vi "RPL_Top_Level_GUI.vi"() -> ()   [LabVIEW 2021]
uses:
  <vilib>/Utility/file.llb/Read Delimited Spreadsheet (string).vi
panel:
  out "Array":string[][](array[string])
  out "subarray":string[](array[string])
  in  "?":bool
  in  "Absolute Change":dbl
  out "ABORT\nACTIVATED":bool
  out "% Change":dbl[](array[numeric])
  in  "% Change":dbl
  out "all rows 2":string[][](array[string])
  in  "Fire Button":bool
  out "IGNITION":bool
  out "DEADMAN\nSWITCH":bool
  in  "Arm Button":bool
  out "POWER DISCONNECTED":bool
  in  "?":bool
  in  "SV6":bool
  in  "SV5":bool
  in  "SV4":bool
  in  "?":bool
  in  "SV3":bool
  in  "SV2":bool
  in  "SV1":bool
  in  "SV0":bool
  in  "GUITabs":T1(tab) caption="Tab Control"
  in  "Deadman Switch Pin":u16(ring) items=["FIO0", "FIO1", "FIO2", "FIO3", "FIO4", "FIO5", "FIO6", "FIO7", "EIO0", "EIO1", "EIO2", "EIO3", "EIO4", "EIO5", "EIO6", "EIO7", "CIO0", "CIO1", "CIO2", "CIO3", "MIO0", "MIO1", "MIO2"]
  in  "Solenoid Supply Pin":u16=5
  in  "LabJack Supply Pin":u16=7
  in  "Relay Supply Pin":u16=9
  in  "Igniter Pin":u16(ring)=7 items=["FIO0", "FIO1", "FIO2", "FIO3", "FIO4", "FIO5", "FIO6", "FIO7", "EIO0", "EIO1", "EIO2", "EIO3", "EIO4", "EIO5", "EIO6", "EIO7", "CIO0", "CIO1", "CIO2", "CIO3", "MIO0", "MIO1", "MIO2"]
  in  "LabJack IP Address":string="192.168.1.199"
  in  "LabJack Connection Type":u16(ring) items=["USB", "Ethernet"]
  in  "S: NO/NC":bool=TRUE
  in  "SV0 Pin":u16(ring)=8 items=["FIO0", "FIO1", "FIO2", "FIO3", "FIO4", "FIO5", "FIO6", "FIO7", "EIO0", "EIO1", "EIO2", "EIO3", "EIO4", "EIO5", "EIO6", "EIO7", "CIO0", "CIO1", "CIO2", "CIO3", "MIO0", "MIO1", "MIO2"]
  in  "SV1 Pin":u16(ring)=9 items=["FIO0", "FIO1", "FIO2", "FIO3", "FIO4", "FIO5", "FIO6", "FIO7", "EIO0", "EIO1", "EIO2", "EIO3", "EIO4", "EIO5", "EIO6", "EIO7", "CIO0", "CIO1", "CIO2", "CIO3", "MIO0", "MIO1", "MIO2"]
  in  "SV3 Pin":u16(ring)=11 items=["FIO0", "FIO1", "FIO2", "FIO3", "FIO4", "FIO5", "FIO6", "FIO7", "EIO0", "EIO1", "EIO2", "EIO3", "EIO4", "EIO5", "EIO6", "EIO7", "CIO0", "CIO1", "CIO2", "CIO3", "MIO0", "MIO1", "MIO2"]
  in  "SV2 Pin":u16(ring)=10 items=["FIO0", "FIO1", "FIO2", "FIO3", "FIO4", "FIO5", "FIO6", "FIO7", "EIO0", "EIO1", "EIO2", "EIO3", "EIO4", "EIO5", "EIO6", "EIO7", "CIO0", "CIO1", "CIO2", "CIO3", "MIO0", "MIO1", "MIO2"]
  in  "SV6 Pin":u16(ring)=14 items=["FIO0", "FIO1", "FIO2", "FIO3", "FIO4", "FIO5", "FIO6", "FIO7", "EIO0", "EIO1", "EIO2", "EIO3", "EIO4", "EIO5", "EIO6", "EIO7", "CIO0", "CIO1", "CIO2", "CIO3", "MIO0", "MIO1", "MIO2"]
  in  "SV5 Pin":u16(ring)=13 items=["FIO0", "FIO1", "FIO2", "FIO3", "FIO4", "FIO5", "FIO6", "FIO7", "EIO0", "EIO1", "EIO2", "EIO3", "EIO4", "EIO5", "EIO6", "EIO7", "CIO0", "CIO1", "CIO2", "CIO3", "MIO0", "MIO1", "MIO2"]
  in  "SV4 Pin":u16(ring)=12 items=["FIO0", "FIO1", "FIO2", "FIO3", "FIO4", "FIO5", "FIO6", "FIO7", "EIO0", "EIO1", "EIO2", "EIO3", "EIO4", "EIO5", "EIO6", "EIO7", "CIO0", "CIO1", "CIO2", "CIO3", "MIO0", "MIO1", "MIO2"]
  in  "S: NO/NC":bool=TRUE
  in  "S: NO/NC":bool=TRUE
  in  "S: NO/NC":bool=TRUE
  in  "S: NO/NC":bool=TRUE
  in  "S: NO/NC":bool=TRUE
  in  "S: NO/NC":bool=TRUE
  in  "R: NC/NO":bool=TRUE
  in  "R: NC/NO":bool=TRUE
  in  "R: NC/NO":bool=TRUE
  in  "R: NC/NO":bool=TRUE
  in  "R: NC/NO":bool=TRUE
  in  "R: NC/NO":bool=TRUE
  in  "R: NC/NO":bool=TRUE
  in  "TC1 Type":u16(ring)=7 items=["B", "E", "J", "K", "N", "R", "S", "T"]
  in  "TC2 Type":u16(ring)=3 items=["B", "E", "J", "K", "N", "R", "S", "T"]
  in  "TC1 +Channel":u16
  in  "TC2 -Channel":u16=3
  in  "TC2 +Channel":u16=2
  in  "TC1 -Channel":u16=1
  in  "PT2 Pin":u16=6
  in  "PT1 Pin":u16=8
  in  "PT3 Pin":u16=4
  in  "LP1 Pin":u16=10
  in  "k [N/m]":dbl=2000.0
  out "?":u32[](array[numeric])
  out "?":bool[](array[boolean])
  out "?":string[](array[string])
  in  "SV0":bool
  out "?":bool[](array[boolean])
  out "?":bool[](array[boolean])
  out "?":bool[](array[boolean])
  in  "SV1":bool
  in  "SV2":bool
  in  "SV3":bool
  out "?":bool[](array[boolean])
  in  "SV4":bool
  out "?":bool[](array[boolean])
  out "?":bool[](array[boolean])
  in  "SV5":bool
  in  "SV6":bool
  in  "Procedure Name":string
  in  "P#":u32
  in  "Add Procedure":bool
  in  "Remove Procedure":bool
  in  "Row":u32
  out "?":u32[](array[numeric])
  out "File Path":path[](array[path])
  out "?":bool
  out "?":bool
  out "?":bool
  out "?":bool
  out "?":bool
  out "?":bool
  out "?":bool
  out "?":bool
  out "?":bool
  out "?":bool
  out "?":bool
  out "?":bool
  out "?":bool
  in  "Dry Test-Run":bool
  out "LabJack Supply Voltage":dbl(slide) scale=0.0..5.0
  out "Solenoid Supply Voltage":dbl(slide) scale=0.0..14.0
  out "Relay Supply Voltage":dbl(slide) scale=0.0..5.0
  out "?":bool
  out "?":bool
  out "?":bool
  out "PT3: Chamber Pressure [psi]":dbl(knob) scale=0.0..500.0
  out "TC1: N2O Temp [°C]":dbl(slide) scale=-20.0..20.0
  out "TC2: Chamber Temp [°C]":dbl(slide) scale=-270.0..1260.0
  out "LP1: Thrust Reading [N]":dbl(slide) scale=0.0..250.0
  out "PT1: N2O Pressure [psi]":dbl(knob) scale=0.0..1000.0
  out "PT2: Ethanol Pressure [psi]":dbl(knob) scale=0.0..1000.0
  out "?":bool
  out "?":bool
  out "?":dbl[][](graph)
  in  "DATA LOGGING":bool
  in  "?":bool
  in  "?":bool
  # "SYSTEM FIRE OPERATION"
  # "CONTROL & ABORT STATUS"
  # "FEED SYSTEM SETTINGS"
  # "HIL TEST PARAMETERS"
  # "THERMOCOUPLE SETTINGS"
  # "SOLENOID VALVE & RELAY SETTINGS"
  # "CALIBRATION SETTINGS"
  # "POWER SYSTEM SETTINGS"
  # "THRUST MEASUREMENT SETTINGS"
  # "LINE & CHAMBER STATUS"
  # "RUNTANK FLOWRATE STATUS"
  # "DATA LOGGING"
  # "POWER SUPPLY STATUS"
  # "THRUST STATUS"
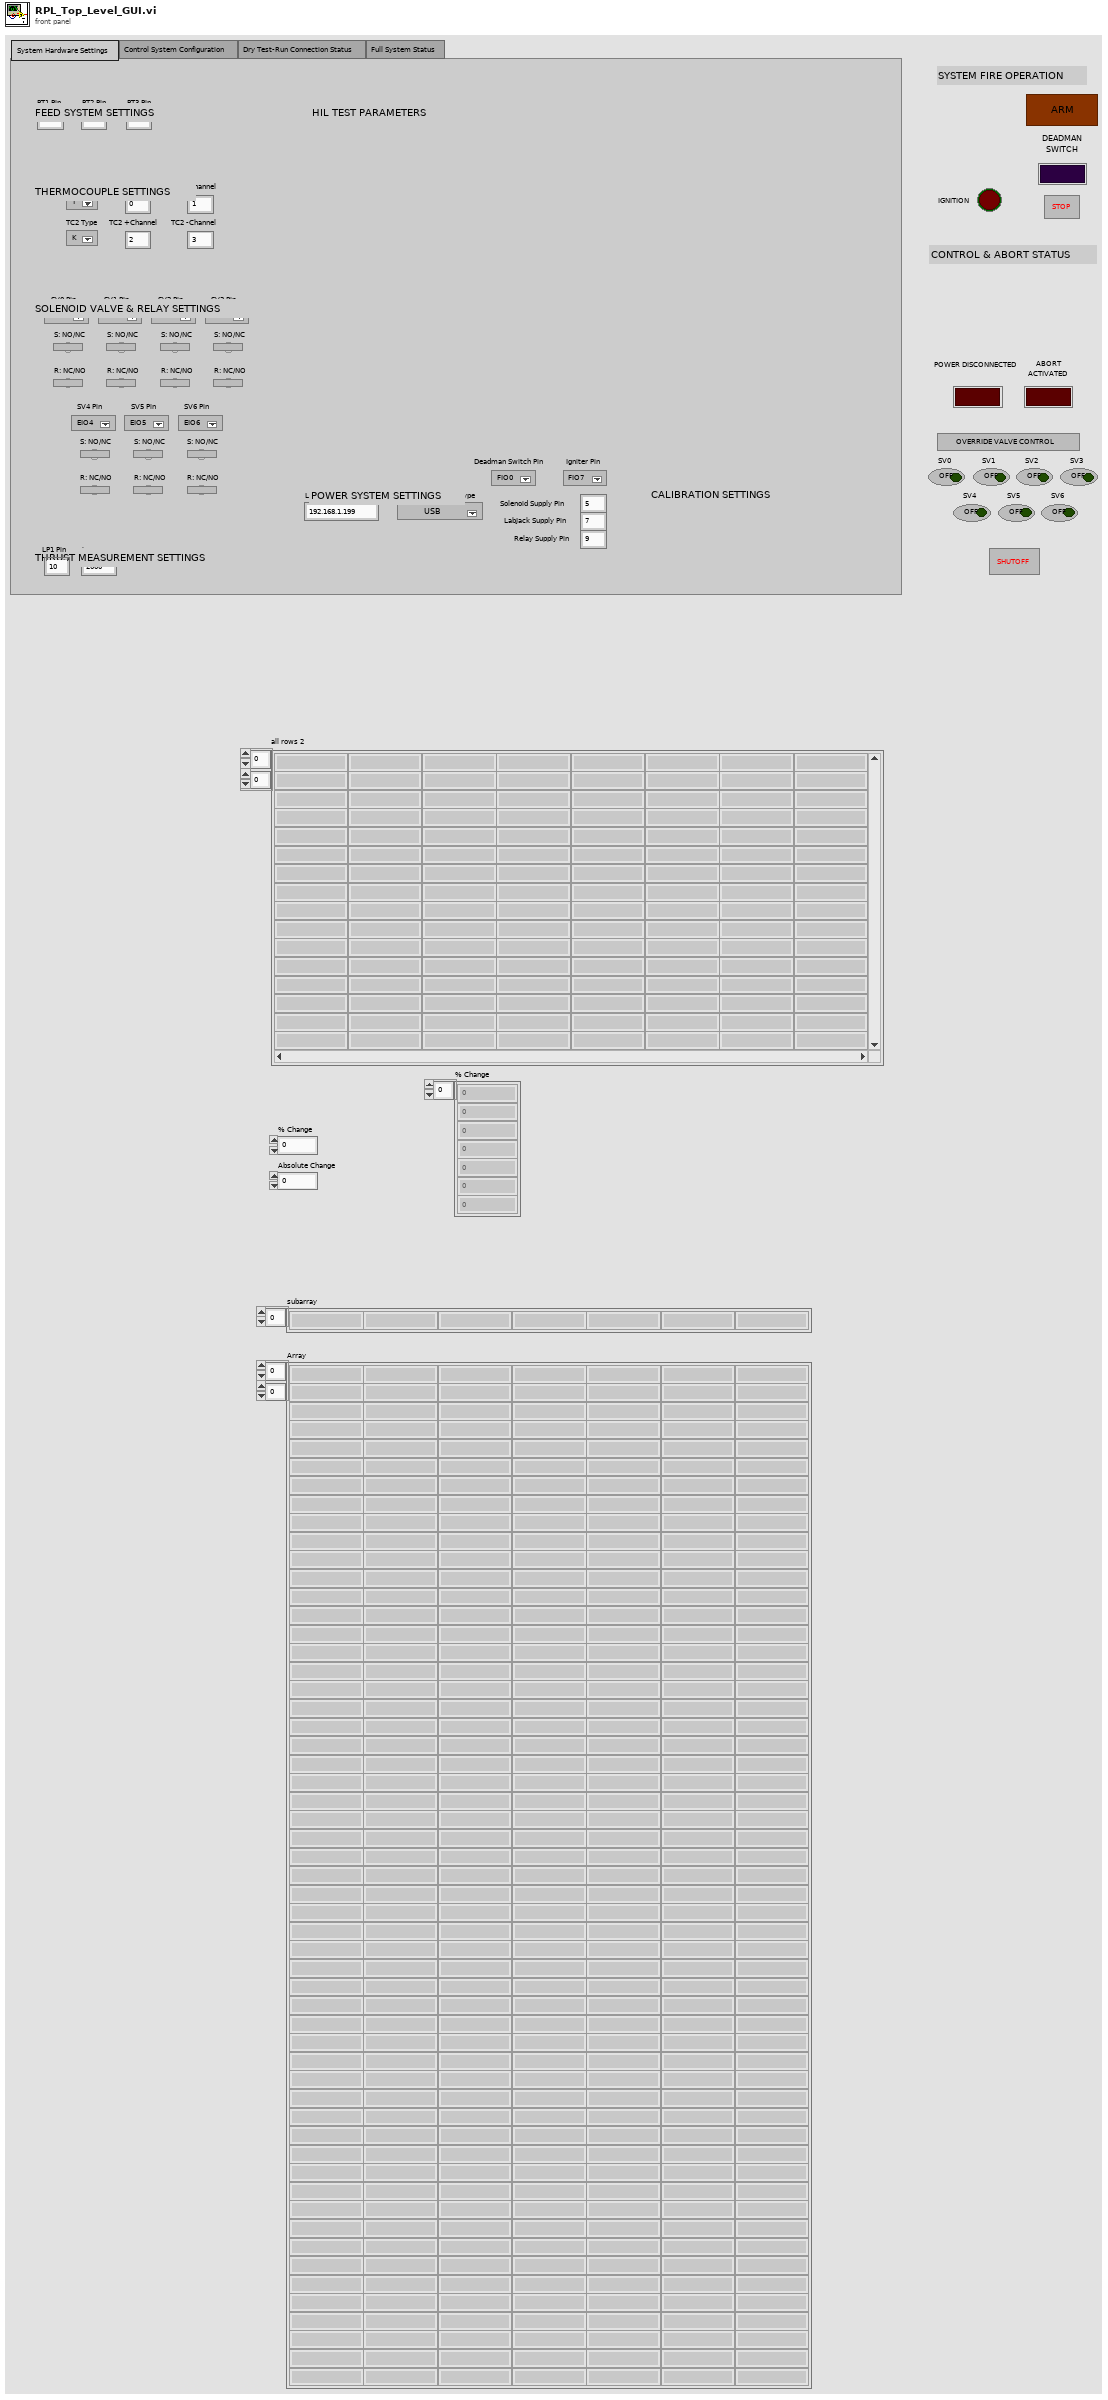
[diagram p1: front panel]
types:
  T1 = enum32{"System Hardware Settings", "Control System Configuration", "Dry Test-Run Connection Status", "Full System Status"}
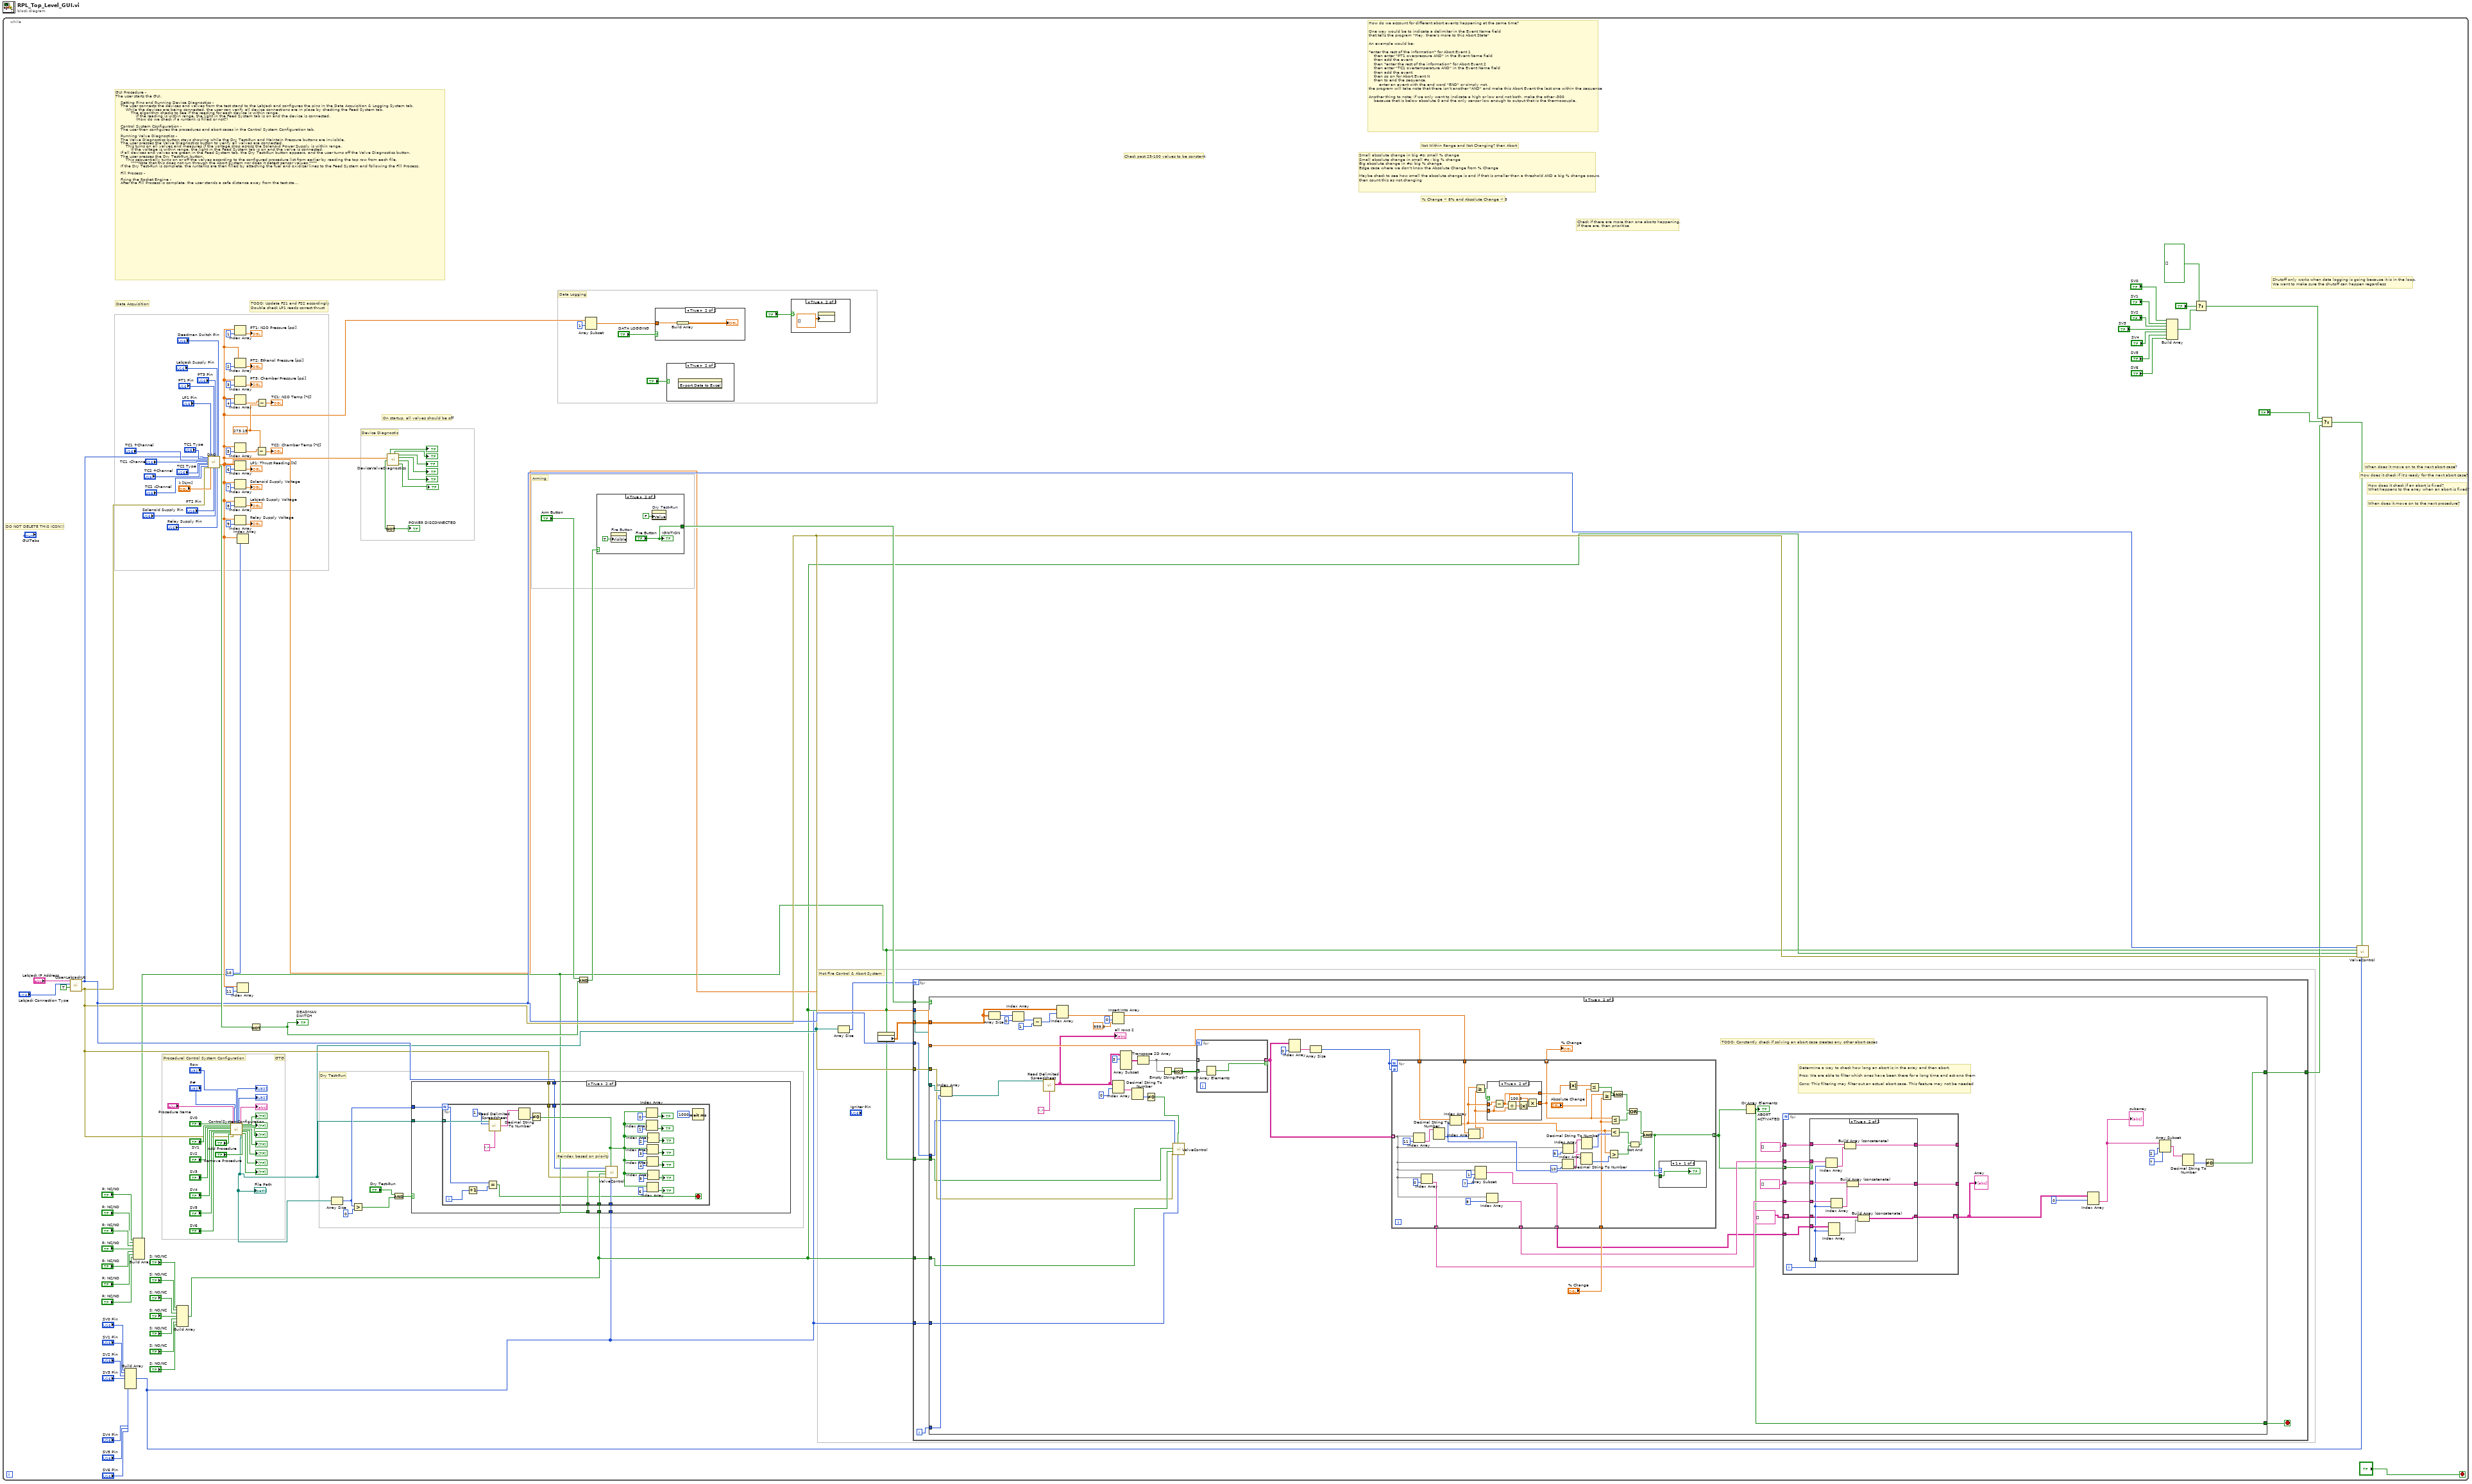
[diagram p0: block diagram]
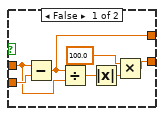
[diagram p4: hidden frame]
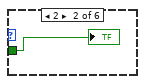
[diagram p5: hidden frame]
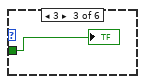
[diagram p6: hidden frame]
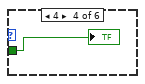
[diagram p7: hidden frame]
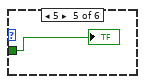
[diagram p8: hidden frame]
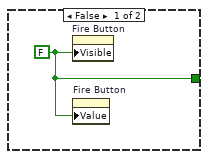
[diagram p13: hidden frame]
diagram:
  n1 = while {
    stop <- "?" stop-if-true
    w30 = 273.15 ("x")
    # "Shutoff only works when data logging is going because it is in the loop.\nWe want to make sure the shutoff can happen regardless"
    # "On startup, all valves should be off"
    # "How does it check if an abort is fixed?\nWhat happens to the array when an abort is fixed?"
    # "How does it check if it's ready for the next abort case?"
    # "When does it move on to the next abort case?"
    # "When does it move on to the next procedure?"
    # "% Change < 8% and Absolute Change < 5"
    # "Small absolute change in big #s: small % change\nSmall absolute change in small #s : big % change\nBig absolute change in #s: big % change\nEdge case where we don't know the Absolute Change from % Change\n\nMaybe check to see how small the absolute change is and if that is smaller than a threshold AND a big % change occurs,\nthen count this as not changing"
    # "Check if there are more than one aborts happening.\nIf there are, then prioritize"
    # "Check past 25-100 values to be constant"
    # "Not Within Range and Not Changing? then Abort"
    # "How do we account for different abort events happening at the same time?\n\nOne way would be to indicate a delimiter in the Event Name field\nthat tells the program \"Hey, there's more to this Abort State\"\n\nAn example would be:\n\n*enter the rest of the information* for Abort Event 1\n    then enter \"PT1 overpressure AND\" in the Event Name field\n    then add the event\n    then *enter the rest of the information* for Abort Event 2\n    then enter \"TC1 overtemperature AND\" in the Event Name field\n    then add the event\n    then so on for Abort Event N\n    then to end the sequence,\n        enter an event with the end word \"END\" or simply not,\nthe program will take note that there isn't another \"AND\" and make this Abort Event the last one within the sequence\n\nAnother thing to note: if we only want to indicate a high or low and not both, make the other -300\n    because that is below absolute 0 and the only sensor low enough to output that is the thermocouple."
    # "DO NOT DELETE THIS ICON!!!"
    # "GUI Procedure -\nThe user starts the GUI.\n\n    Setting Pins and Running Device Diagnostics -\n    The user connects the devices and valves from the test stand to the LabJack and configures the pins in the Data Acquisition & Logging System tab.\n        While the devices are being connected, the user can verify all device connections are in place by checking the Feed System tab.\n            The algorithm checks to see if the reading for each device is within range.\n                If the reading is within range, the light in the Feed System tab is on and the device is connected.\n                (How do we check if a runtank is filled or not?)\n\n    Control System Configuration -\n    The user then configures the procedures and abort cases in the Control System Configuration tab.\n\n    Running Valve Diagnostics -\n    The Valve Diagnostics button stays showing while the Dry Test-Run and Maintain Pressure buttons are invisible.\n    The user presses the Valve Diagnostics button to verify all valves are connected.\n        This turns on all valves and measures if the voltage drop across the Solenoid Power Supply is within range.\n            If the voltage is within range, the light in the Feed System tab is on and the valve is connected.\n    If all devices and valves are green in the Feed System tab, the Dry Test-Run button appears, and the user turns off the Valve Diagnostics button.\n    The user presses the Dry Test-Run button.\n        This sequentially turns on or off the valves according to the configured procedure list from earlier by reading the top row from each file.\n            ****Note that this does not run through the Abort System nor does it detect sensor values.****\n    If the Dry Test-Run is complete, the runtanks are then filled by attaching the fuel and oxidizer lines to the Feed System and following the Fill Process.\n\n    Fill Process -\n\n    Firing the Rocket Engine -\n    After the Fill Process is complete, the user stands a safe distance away from the test stand.\n    The runtanks are massed to check if they are filled.\n        This makes the Maintain Pressure button appear and makes the Valve Diagnostics button and the Dry Test-Run button invisible and off to avoid further misclicking.\n    The user presses the Maintain Pressure button to not let the Feed System depressurize. The rocket engine is ready to fire.\n    To fire the rocket engine, the user presses the Arm button [on the count of 3] and holds down the Deadman Switch [on the count of 2].\n        This makes the Fire button appear and makes the Maintain Pressure button invisible and off to avoid further misclicking.\n        The user presses the Fire button [on the count of 1] to fire the rocket engine."
    # "Hot Fire Control & Abort System"
    # "Data Logging"
    # "Arming"
    # "Dry Test-Run"
    # "Device Diagnostic"
    # "TODO: Update FS1 and FS2 accordingly\nDouble check LP1 reads correct thrust"
    # "Data Acquisition"
    # "GTG"
    # "Procedural Control System Configuration"
    n2 = call "OpenLabJackU6.vi"("Select First Found"=TRUE, "Connection Type"="LabJack Connection Type", "U6 Address"="LabJack IP Address") -> ("error out"=w10:errorcluster, "Handle"=w11:i32)  [unwired: 1 in, 1 out]
    n3 = Build Array("SV0 Pin", "SV1 Pin", "SV2 Pin", "SV3 Pin", "SV4 Pin", "SV5 Pin", "SV6 Pin") -> (w1:u16[])
    n4 = Build Array("R: NC/NO", "R: NC/NO", "R: NC/NO", "R: NC/NO", "R: NC/NO", "R: NC/NO", "R: NC/NO") -> (w3:bool[])
    n5 = Build Array("S: NO/NC", "S: NO/NC", "S: NO/NC", "S: NO/NC", "S: NO/NC", "S: NO/NC", "S: NO/NC") -> (w2:bool[])
    n6 = call "DAQ.vi"("Handle In"=w11, "TC1 Type"="TC1 Type", "TC1 +Channel"="TC1 +Channel", "TC1 -Channel"="TC1 -Channel", "TC2 Type"="TC2 Type", "TC2 +Channel"="TC2 +Channel", "TC2 -Channel"="TC2 -Channel", "error in"=w10, "LP1 Pin"="LP1 Pin", "k [N/m]"="k [N/m]", "PT1 Pin"="PT1 Pin", "PT2 Pin"="PT2 Pin", "PT3 Pin"="PT3 Pin", "Solenoid Supply Pin"="Solenoid Supply Pin", "LabJack Supply Pin"="LabJack Supply Pin", "Relay Supply Pin"="Relay Supply Pin", "Deadman Switch Pin"="Deadman Switch Pin") -> ("Sensor Values"=w9:dbl[], "Deadman Switch"=w131:bool)  [unwired: 8 in, 1 out]
    n7 = call "ControlSystemConfiguration.vi"("SV0"="SV0", "SV1"="SV1", "SV2"="SV2", "SV3"="SV3", "SV4"="SV4", "SV5"="SV5", "SV6"="SV6", "Add Procedure"="Add Procedure", "Procedure Name"="Procedure Name", "error in"=w10, "P#"="P#", "Row"="Row", "Remove Procedure"="Remove Procedure") -> ("Row"=→"?":u32[], 16:→"?":u32[], 18:→"?":string[], "File Path"=w5:path[], 20:→"?":bool[], 21:→"?":bool[], 22:→"?":bool[], 23:→"?":bool[], 24:→"?":bool[], 25:→"?":bool[], 26:→"?":bool[])  [unwired: 3 in, 1 out]
    "File Path" <- w5
    n8 = Index Array(array=w9, index=1) -> (element=→"PT1: N2O Pressure [psi]":dbl)
    n9 = Index Array(array=w9, index=2) -> (element=→"PT2: Ethanol Pressure [psi]":dbl)
    n10 = Index Array(array=w9, index=3) -> (element=→"PT3: Chamber Pressure [psi]":dbl)
    n11 = Index Array(array=w9, index=4) -> (element=w126:dbl)
    n12 = Index Array(array=w9, index=5) -> (element=w127:dbl)
    n13 = Index Array(array=w9, index=6) -> (element=→"LP1: Thrust Reading [N]":dbl)
    n14 = Index Array(array=w9, index=7) -> (element=→"Solenoid Supply Voltage":dbl)
    n15 = Index Array(array=w9, index=8) -> (element=→"LabJack Supply Voltage":dbl)
    n16 = Index Array(array=w9, index=9) -> (element=→"Relay Supply Voltage":dbl)
    n17 = Index Array(array=w9, index=10) -> ()  [unwired: 1 out]
    n18 = Index Array(array=w9, index=11) -> ()  [unwired: 1 out]
    n19 = Not(x=w131) -> (.not. x?=w4:bool)
    "DEADMAN\nSWITCH" <- w4
    n20 = Subtract(x=w127, y=w30) -> (x-y=→"TC2: Chamber Temp [°C]":dbl)
    n21 = Subtract(x=w126, y=w30) -> (x-y=→"TC1: N2O Temp [°C]":dbl)
    n22 = Array Size(array=w5) -> (size(s)=w111:i32)
    n23 = Greater?(x=w111, y=0) -> (0:w108:bool)
    n24 = call "DeviceValveDiagnostics.vi"("Sensor Values"=w9) -> (0:→"?":bool, "Power Connected"=w98:bool, 4:→"?":bool, 6:→"?":bool, 7:→"?":bool, 8:→"?":bool, 9:→"?":bool)  [unwired: 2 out]
    n25 = Not(x=w98) -> (.not. x?=→"POWER DISCONNECTED":bool)
    n26 = And(x="Dry Test-Run", y=w108) -> (x .and. y?=w106:bool)
    n27 = case shown="True" w106 {
      tunnel: w111 -> [_ w294]
      tunnel: w5 -> [_ w293]
      tunnel: w11 -> [_ w292]
      tunnel: w10 -> [_ w291]
      tunnel: w3 -> [_ w290]
      tunnel: w1 -> [_ w289]
      tunnel: w2 -> [_ w288]
      frame False {
      }
      frame True {
        n28 = for {
          N: w294 -> [w296]
          tunnel: w293 -> [w324] mode=indexing
          tunnel: w292 -> [w303]
          tunnel: w291 -> [w302]
          tunnel: w290 -> [w301]
          tunnel: w289 -> [w300]
          tunnel: w288 -> [w299]
          i -> [w297]
          stop <- w295 stop-if-true
          # "Reindex based on priority"
          n29 = Increment(x=w297) -> (x+1=w298:i32)
          n30 = Equal?(x=w296, y=w298) -> (x = y?=w295:bool)
          n31 = call-poly <vilib>:"Read Delimited Spreadsheet.vi"("file path (dialog if empty)"=w324, "number of rows (all:-1)"=1, "delimiter (\\t)"="," ("delimiter (\\t)")) -> ("first row"=w321:string[])  [unwired: 7 in, 5 out]
          n32 = Decimal String To Number(string=w321) -> (number=w320:i32[])  [unwired: 2 in, 1 out]
          n33 = Not Equal To 0?(x=w320) -> (x != 0?=w304:bool[])
          n34 = call "ValveControl.vi"("SV Pin"=w300, "Solenoid States"=w304, "error in"=w302, "Solenoid NC/NO"=w299, "Relay NO/NC"=w301, "Handle In"=w303) -> ()  [unwired: 1 out]
          n35 = Index Array(array=w304, index=0) -> (element=→"?":bool)
          n36 = Index Array(array=w304, index=1) -> (element=→"?":bool)
          n37 = Index Array(array=w304, index=6) -> (element=→"?":bool)
          n38 = Index Array(array=w304, index=3) -> (element=→"?":bool)
          n39 = Index Array(array=w304, index=4) -> (element=→"?":bool)
          n40 = Index Array(array=w304, index=2) -> (element=→"?":bool)
          n41 = Index Array(array=w304, index=5) -> (element=→"?":bool)
          n42 = Wait (ms)(milliseconds to wait=u32 1000) -> ()  [unwired: 1 out]
        }
      }
    }
    n43 = Compound Arithmetic op=AND("Arm Button", w4) -> (w110:bool)
    n44 = Array Subset(array=w9, index=1) -> (w113:dbl[])  [unwired: 1 in]
    n45 = case shown="True" w110 {
      tunnel: [w284 "Fire Button"] -> w12
      frame False {
        w284 = FALSE ("Visible")
        n46 = property on="Fire Button" class="Bool (strict)"("Visible"=w284) -> ()  [unwired: 2 in, 2 out]
        n47 = property on="Fire Button" class="Bool (strict)"("Value"=w284) -> ()  [unwired: 2 in, 2 out]
      }
      frame True {
        n48 = property on="Fire Button" class="Bool (strict)"("Visible"=TRUE) -> ()  [unwired: 2 in, 2 out]
        n49 = property on="Dry Test-Run" class="Bool (strict)"("Value"=FALSE ("Dry Test-Run")) -> ()  [unwired: 2 in, 2 out]
        "IGNITION" <- "Fire Button"
      }
    }
    n50 = case shown="True" "DATA LOGGING" {
      tunnel: w113 -> [_ w283]
      frame False {
      }
      frame True {
        n51 = Build Array(w283) -> (→"?":dbl[][])
      }
    }
    n52 = case shown="True" "?" {
      frame False {
      }
      frame True {
        n53 = invoke class="WFChart (strict)" method="Export Data to Excel"() -> ()  [unwired: 3 in, 3 out]
      }
    }
    n54 = case shown="True" "?" {
      frame False {
      }
      frame True {
        n55 = property class="WFChart (strict)"("History Data"=dbl[][] []) -> ()  [unwired: 2 in, 2 out]
      }
    }
    n56 = Array Size(array=w5) -> (size(s)=w6:i32)
    n57 = property class="WFChart (strict)"() -> ("History Data"=w8:dbl[][])  [unwired: 2 in, 2 out]
    n58 = for {
      N: w6 -> [_]
      tunnel: w12 -> [w143]
      tunnel: w11 -> [w133]
      tunnel: w10 -> [w142]
      tunnel: w9 -> [w141]
      tunnel: w5 -> [w140]
      tunnel: w3 -> [_]
      tunnel: w2 -> [_]
      tunnel: w1 -> [_]
      tunnel: w8 -> [w139]
      tunnel: [w138] -> w7
      tunnel: w3 -> [w135]
      tunnel: w2 -> [w134]
      tunnel: w1 -> [w132]
      i -> [w137]
      stop <- w136 stop-if-true
      n59 = case shown="True" w143 {
        tunnel: w142 -> [_ w146]
        tunnel: w141 -> [_ w173]
        tunnel: w140 -> [_ w193]
        tunnel: w139 -> [_ w176]
        tunnel: [_ w156] -> w138
        tunnel: w137 -> [_ w155]
        tunnel: [_ w154] -> w136
        tunnel: w135 -> [_ w145]
        tunnel: w134 -> [_ w148]
        tunnel: w133 -> [_ w144]
        tunnel: w132 -> [_ w149]
        frame False {
        }
        frame True {
          # "Determine a way to check how long an abort is in the array and then abort.\n\nPros: We are able to filter which ones have been there for a long time and act ono them\n\nCons: This filtering may filter out an actual abort case. This feature may not be needed"
          # "TODO: Constantly check if solving an abort case creates any other abort cases"
          n60 = Index Array(array=w193, index=w155) -> (element=w195:path)
          n61 = Array Size(array=w176) -> (size(s)=w182:i32[])
          n62 = Index Array(array=w182, index=0) -> (element=w183:i32)
          n63 = Subtract(x=w183, y=1) -> (x-y=w184:i32)
          n64 = call-poly <vilib>:"Read Delimited Spreadsheet.vi"("file path (dialog if empty)"=w195, "delimiter (\\t)"="," ("delimiter (\\t)")) -> ("all rows"=w150:string[][])  [unwired: 8 in, 5 out]
          "all rows 2" <- w150
          n65 = Index Array(array=w176, index (row)=w184) -> (element=w181:dbl[])  [unwired: 1 in]
          n66 = Insert Into Array(array=w181, index=0, new element=999.0 ("new element/subarray")) -> (w172:dbl[])
          n67 = Index Array(array=w150, index (row)=0) -> (element=w152:string[])  [unwired: 1 in]
          n68 = Array Subset(array=w150, index (row)=3 ("index")) -> (w192:string[][])  [unwired: 3 in]
          n69 = Decimal String To Number(string=w152) -> (number=w151:i32[])  [unwired: 2 in, 1 out]
          n70 = Transpose 2D Array(2D array=w192) -> (transposed array=w190:string[][])
          n71 = Not Equal To 0?(x=w151) -> (x != 0?=w147:bool[])
          n72 = Empty String/Path?(string/path=w190) -> (empty?=w191:bool[][])
          n73 = Not(x=w191) -> (.not. x?=w189:bool[][])
          n74 = call "ValveControl.vi"("SV Pin"=w149, "Solenoid States"=w147, "error in"=w146, "Solenoid NC/NO"=w148, "Relay NO/NC"=w145, "Handle In"=w144) -> ()  [unwired: 1 out]
          n75 = for {
            tunnel: w190 -> [w279] mode=indexing
            tunnel: w189 -> [w280] mode=indexing
            tunnel: [w279] -> w187 mode=indexing if=w278
            n76 = Or Array Elements(Boolean array=w280) -> (logical OR=w278:bool)
          }
          n77 = Index Array(array=w187, index (col)=0 ("disabled index (col)")) -> (element=w186:string[])  [unwired: 1 in]
          n78 = Array Size(array=w186) -> (size(s)=w174:i32)
          n79 = for {
            N: w174 -> [_]
            tunnel: w187 -> [w242] mode=indexing
            tunnel: w173 -> [w256]
            tunnel: w172 -> [w255]
            tunnel: "% Change" -> [w225]
            workers-P: w174 -> [_]
            tunnel: [w226] -> w175 mode=indexing
            tunnel: [w241] -> w164 mode=indexing
            tunnel: [w245] -> w169 mode=indexing
            tunnel: [w240] -> w170 mode=indexing
            tunnel: [w239] -> w168 mode=indexing
            n80 = Index Array(array=w242, index=11) -> (element=w257:string)
            n81 = Index Array(array=w242, index=0) -> (element=w245:string)
            n82 = Decimal String To Number(string=w257) -> (number=w244:i32)  [unwired: 2 in, 1 out]
            n83 = Index Array(array=w256, index=w244) -> (element=w234:dbl)
            n84 = Index Array(array=w255, index=w244) -> (element=w233:dbl)
            n85 = Greater Or Equal?(x=w234, y=w233) -> (x >= y?=w235:bool)
            n86 = Array Subset(array=w242, index=1, length=7) -> (w239:string[])
            n87 = Index Array(array=w242, index=8) -> (element=w240:string)
            n88 = case shown="True" w235 {
              tunnel: w234 -> [w261 w272]
              tunnel: w233 -> [w262 w271]
              tunnel: [w260 w267] -> w226
              tunnel: [w259 w266] -> w230
              frame False {
                n89 = Subtract(x=w261, y=w262) -> (x-y=w259:dbl)
                n90 = Divide(x=w259, y=w261) -> (x/y=w265:dbl)
                n91 = Absolute Value(x=w265) -> (abs(x)=w264:dbl)
                n92 = Multiply(x=100.0, y=w264) -> (x*y=w260:dbl)
              }
              frame True {
                n93 = Subtract(x=w272, y=w271) -> (x-y=w266:dbl)
                n94 = Divide(x=w266, y=w271) -> (x/y=w270:dbl)
                n95 = Absolute Value(x=w270) -> (abs(x)=w269:dbl)
                n96 = Multiply(x=100.0, y=w269) -> (x*y=w267:dbl)
              }
            }
            n97 = Index Array(array=w242, index=10) -> (element=w251:string)
            n98 = Index Array(array=w242, index=9) -> (element=w253:string)
            n99 = Absolute Value(x=w230) -> (abs(x)=w223:dbl)
            n100 = Decimal String To Number(string=w251) -> (number=w249:i32)  [unwired: 2 in, 1 out]
            n101 = Decimal String To Number(string=w253) -> (number=w250:i32)  [unwired: 2 in, 1 out]
            n102 = Less Or Equal?(x=w223, y="Absolute Change") -> (x <= y?=w228:bool)
            n103 = Greater Or Equal?(x=w226, y=w225) -> (x >= y?=w227:bool)
            n104 = Greater?(x=w234, y=w249) -> (0:w237:bool)
            n105 = Less?(x=w234, y=w250) -> (x < y?=w238:bool)
            n106 = Less Or Equal?(x=w226, y=w225) -> (x <= y?=w232:bool)
            n107 = And(x=w228, y=w227) -> (x .and. y?=w224:bool)
            n108 = Or(x=w224, y=w232) -> (x .or. y?=w231:bool)
            n109 = Not And(1:w237, 2:w238) -> (0:w236:bool)
            n110 = And(x=w231, y=w236) -> (x .and. y?=w241:bool)
            n111 = case shown="1" w244 {
              tunnel: w241 -> [w273 w274 w275 w276 w277 _]
              frame 1 {
                "?" <- w273
              }
              frame 2 {
                "?" <- w274
              }
              frame 3 {
                "?" <- w275
              }
              frame 4 {
                "?" <- w276
              }
              frame 5 {
                "?" <- w277
              }
              frame 0, Default {
              }
            }
          }
          "% Change" <- w175
          n112 = Or Array Elements(Boolean array=w164) -> (logical OR=w154:bool)
          "ABORT\nACTIVATED" <- w154
          n113 = for {
            tunnel: w164 -> [w197] mode=indexing
            tunnel: w170 -> [w205]
            tunnel: w169 -> [w204]
            tunnel: w168 -> [w199]
            tunnel: string[] [] ("sorted array") -> [w200]
            tunnel: [w201] -> _
            tunnel: string[] [] ("sorted array") -> [w202]
            tunnel: [w203] -> _
            shift-right: [w198] -> w158
            shift-left: string[][] [] -> [w196]
            i -> [w206]
            n114 = case shown="True" w197 {
              tunnel: w202 -> [w209 w222]
              tunnel: w206 -> [_ w212]
              tunnel: w205 -> [_ w221]
              tunnel: w200 -> [w208 w219]
              tunnel: w204 -> [_ w218]
              tunnel: [w209 w216] -> w203
              tunnel: [w208 w215] -> w201
              tunnel: w199 -> [_ w213]
              tunnel: [w207 w210] -> w198
              tunnel: w196 -> [w207 w211]
              frame False {
              }
              frame True {
                n115 = Index Array(array=w221, index=w212) -> (element=w217:string)
                n116 = Index Array(array=w213, index (row)=w212) -> (element=w214:string[])  [unwired: 1 in]
                n117 = Index Array(array=w218, index=w212) -> (element=w220:string)
                n118 = Build Array (concatenate)(w222, w217) -> (w216:string[])
                n119 = Build Array (concatenate)(w219, w220) -> (w215:string[])
                n120 = Build Array (concatenate)(w211, w214) -> (w210:string[][])
              }
            }
          }
          "Array" <- w158
          n121 = Index Array(array=w158, index (row)=0) -> (element=w163:string[])  [unwired: 1 in]
          "subarray" <- w163
          n122 = Array Subset(array=w163, index=2, length=7) -> (w162:string[])
          n123 = Decimal String To Number(string=w162) -> (number=w161:i32[])  [unwired: 2 in, 1 out]
          n124 = Not Equal To 0?(x=w161) -> (x != 0?=w156:bool[])
        }
      }
    }
    n125 = Build Array("SV0", "SV1", "SV2", "SV3", "SV4", "SV5", "SV6") -> (w129:bool[])
    n126 = Select(t=bool[] [], s="?", f=w129) -> (s? t:f=w130:bool[])
    n127 = Select(t=w130, s="?", f=w7) -> (s? t:f=w13:bool[])
    n128 = call "ValveControl.vi"("SV Pin"=w1, "Solenoid States"=w13, "error in"=w10, "Solenoid NC/NO"=w2, "Relay NO/NC"=w3, "Handle In"=w11) -> ()  [unwired: 1 out]
  }
